vi "Initialize Menus and SVs.vi"(8 "error in":errorcluster, 11 "Menu in":refnum<k9>) -> (0 "error out":errorcluster)   [LabVIEW 2012]
uses:
  <userlib>/_JGCODE/error_logger/_error_logger.llb/ErrorLogger.lvclass
  Reusable/File IO/File Utilities.lvlib
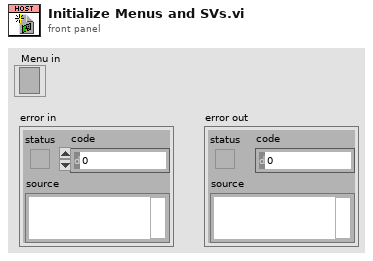
[diagram p1: front panel]
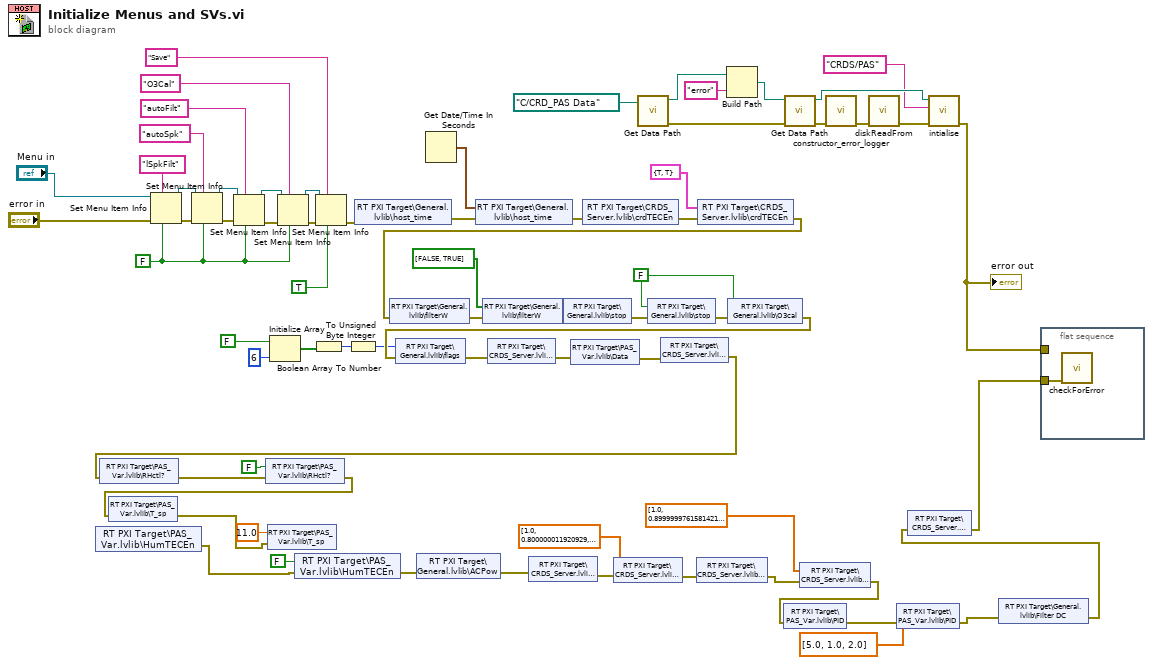
[diagram p0: block diagram]
diagram:
  w55 = FALSE ("stop")
  w21 = FALSE ("checked")
  n1 = shared-variable "RT PXI Target\\PAS_Var.lvlib\\HumTECEn"() -> (error out=w45:errorcluster)  [unwired: 1 in, 1 out]
  n2 = Set Menu Item Info(6:w21, 7:"lSpkFilt" ("item tag"), 8:"error in", 11:"Menu in") -> (0:w59:errorcluster, 3:w60:refnum<k9>)  [unwired: 3 in]
  n3 = Set Menu Item Info(6:w21, 7:"autoSpk" ("item tag"), 8:w59, 11:w60) -> (0:w63:errorcluster, 3:w62:refnum<k9>)  [unwired: 3 in]
  n4 = Set Menu Item Info(6:w21, 7:"autoFilt" ("item tag"), 8:w63, 11:w62) -> (0:w66:errorcluster, 3:w65:refnum<k9>)  [unwired: 3 in]
  n5 = Initialize Array(FALSE, 6 ("dimension size")) -> (w24:bool[])
  n6 = Set Menu Item Info(6:w21, 7:"O3Cal" ("item tag"), 8:w66, 11:w65) -> (0:w69:errorcluster, 3:w70:refnum<k9>)  [unwired: 3 in]
  n7 = shared-variable "RT PXI Target\\PAS_Var.lvlib\\HumTECEn"(FALSE ("HumTECEn"), error in=w45) -> (error out=w34:errorcluster)
  n8 = Boolean Array To Number(Boolean array=w24) -> (number=w23:u32)
  n9 = Set Menu Item Info(6:TRUE ("checked"), 7:"Save" ("item tag"), 8:w69, 11:w70) -> (0:w41:errorcluster)  [unwired: 3 in, 1 out]
  n10 = To Unsigned Byte Integer(number=w23) -> (unsigned 8bit integer=w22:u8)
  n11 = shared-variable "RT PXI Target\\General.lvlib\\host_time"(error in=w41) -> (error out=w40:errorcluster)  [unwired: 1 out]
  n12 = shared-variable "RT PXI Target\\General.lvlib\\ACPow"(error in=w34) -> (error out=w32:errorcluster)  [unwired: 1 out]
  n13 = Get Date/Time In Seconds() -> (seconds since 1Jan1904=w50:timestamp)
  n14 = shared-variable "RT PXI Target\\General.lvlib\\host_time"(w50, error in=w40) -> (error out=w39:errorcluster)
  n15 = shared-variable "RT PXI Target\\CRDS_Server.lvlib\\Med"(error in=w32) -> (error out=w31:errorcluster)  [unwired: 1 out]
  n16 = shared-variable "RT PXI Target\\CRDS_Server.lvlib\\crdTECEn"(error in=w39) -> (error out=w38:errorcluster)  [unwired: 1 out]
  n17 = shared-variable "RT PXI Target\\CRDS_Server.lvlib\\Med"(sgl[] [1.0, 0.8, 10.0] ("Med"), error in=w31) -> (error out=w30:errorcluster)
  n18 = call "Get Data Path.vi"("Data Path In"=path "C:/CRD_PAS Data" ("Data Path")) -> ("error out"=w11:errorcluster, "Data Path Out"=w5:path)  [unwired: 9 in]
  n19 = shared-variable "RT PXI Target\\CRDS_Server.lvlib\\High"(error in=w30) -> (error out=w29:errorcluster)  [unwired: 1 out]
  n20 = shared-variable "RT PXI Target\\CRDS_Server.lvlib\\crdTECEn"(cluster{"med":bool, "high":bool} {"med"=TRUE, "high"=TRUE} ("crdTECEn"), error in=w38) -> (error out=w17:errorcluster)
  n21 = shared-variable "RT PXI Target\\General.lvlib\\filterW"(error in=w17) -> (error out=w56:errorcluster)  [unwired: 1 out]
  n22 = shared-variable "RT PXI Target\\General.lvlib\\filterW"(bool[] [FALSE, TRUE] ("filterW"), error in=w56) -> (error out=w51:errorcluster)
  n23 = shared-variable "RT PXI Target\\General.lvlib\\stop"(error in=w51) -> (error out=w54:errorcluster)  [unwired: 1 out]
  n24 = shared-variable "RT PXI Target\\General.lvlib\\stop"(w55, error in=w54) -> (error out=w53:errorcluster)
  n25 = Build Path(base path=w5, name or relative path="error") -> (appended path=w12:path)
  n26 = shared-variable "RT PXI Target\\General.lvlib\\O3cal"(w55, error in=w53) -> (error out=w27:errorcluster)
  n27 = shared-variable "RT PXI Target\\General.lvlib\\flags"(w22, error in=w27) -> (error out=w52:errorcluster)
  n28 = shared-variable "RT PXI Target\\CRDS_Server.lvlib\\data"(error in=w52) -> (error out=w37:errorcluster)  [unwired: 1 out]
  n29 = shared-variable "RT PXI Target\\PAS_Var.lvlib\\Data"(error in=w37) -> (error out=w36:errorcluster)  [unwired: 1 out]
  n30 = shared-variable "RT PXI Target\\CRDS_Server.lvlib\\flow"(error in=w36) -> (error out=w35:errorcluster)  [unwired: 1 out]
  n31 = shared-variable "RT PXI Target\\PAS_Var.lvlib\\RHctl?"(error in=w35) -> (error out=w47:errorcluster)  [unwired: 1 out]
  n32 = shared-variable "RT PXI Target\\PAS_Var.lvlib\\RHctl?"(FALSE ("RHctl?"), error in=w47) -> (error out=w48:errorcluster)
  n33 = shared-variable "RT PXI Target\\PAS_Var.lvlib\\T_sp"(error in=w48) -> (error out=w46:errorcluster)  [unwired: 1 out]
  n34 = shared-variable "RT PXI Target\\PAS_Var.lvlib\\T_sp"(sgl 11.0 ("T_sp"), error in=w46) -> ()  [unwired: 1 out]
  n35 = call "Get Data Path.vi"("error in"=w11, "Data Path In"=w12) -> ("error out"=w10:errorcluster, "Data Path Out"=w9:path)  [unwired: 8 in]
  n36 = shared-variable "RT PXI Target\\CRDS_Server.lvlib\\High"(sgl[] [1.0, 0.9, 10.0] ("Med"), error in=w29) -> (error out=w18:errorcluster)
  n37 = shared-variable "RT PXI Target\\PAS_Var.lvlib\\PID"(error in=w18) -> (error out=w20:errorcluster)  [unwired: 1 out]
  n38 = call <userlib>:"constructor_error_logger.vi"("error in (no error)"=w10) -> ("error out"=w16:errorcluster)  [unwired: 10 in]
  n39 = call <userlib>:"diskReadFrom.vi"("error in (no error)"=w16) -> ("error out"=w15:errorcluster)  [unwired: 10 in]
  n40 = shared-variable "RT PXI Target\\PAS_Var.lvlib\\PID"(sgl[] [5.0, 1.0, 2.0] ("PID"), error in=w20) -> (error out=w2:errorcluster)
  n41 = call <userlib>:"intialise.vi"("error in (no error)"=w15, "Application Name (Application)"="CRDS/PAS", "Error Log Folder"=w9) -> ("error out"=w7:errorcluster)  [unwired: 7 in, 1 out]
  "error out" <- w7
  n42 = shared-variable "RT PXI Target\\General.lvlib\\Filter DC"(error in=w2) -> (error out=w1:errorcluster)  [unwired: 1 out]
  n43 = shared-variable "RT PXI Target\\CRDS_Server.lvlib\\Tsp"(error in=w1) -> (error out=w6:errorcluster)  [unwired: 1 out]
  n44 = flat-sequence {
    tunnel: w7 -> [_]
    tunnel: w6 -> [w72]
    frame #0 {
      n45 = call <userlib>:"checkForError.vi"("Error In"=w72) -> ()  [unwired: 9 in, 2 out]
    }
  }
